vi "Hide Info.vi"(7 "Action? (T) in":bool=TRUE, 10 "Hide in":bool, 11 "Game Board in":refnum<class "Game Board.lvclass">) -> ()   [LabVIEW 2021, in "Game Board.lvclass"]
doc: "MIT Licence\nCopyright (c) 2024 David Grollier"
uses:
  Game Board.lvclass
  Game Board.lvclass/Game Board.ctl
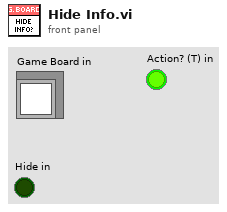
[diagram p1: front panel]
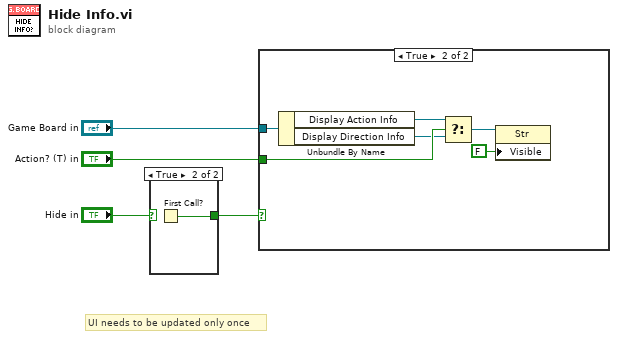
[diagram p0: block diagram]
diagram:
  # "UI needs to be updated only once"
  n1 = case shown="True" "Hide in" {
    selector: "Hide in" -> [w5 _]
    tunnel: [w5 w6] -> w1
    frame False {
    }
    frame True {
      n2 = First Call?() -> (First Call?: T/F=w6:bool)
    }
  }
  n3 = case shown="True" w1 {
    tunnel: "Game Board in" -> [_ w12]
    tunnel: "Action? (T) in" -> [_ w11]
    frame False {
    }
    frame True {
      n4 = Unbundle By Name(w12) -> ("Display Action Info"=w10:refnum<vi>, "Display Direction Info"=w9:refnum<vi>)
      n5 = Select(t=w10, s=w11, f=w9) -> (s? t:f=w8:refnum<vi>)
      n6 = property class="Str"(reference=w8, "Visible"=FALSE) -> ()  [unwired: 1 in, 2 out]
    }
  }
